vi "DateTimeStringToTimeString.vi"(10 "input string":string) -> (2 "concatenated string":string)   [LabVIEW 2012]
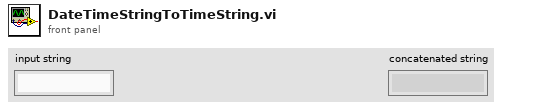
[diagram p1: front panel]
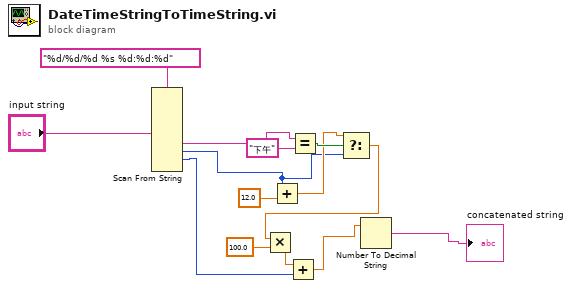
[diagram p0: block diagram]
diagram:
  n1 = Scan From String(format string="%d/%d/%d %s %d:%d:%d", input string="input string") -> (output 4=w12:string, output 5=w7:i32, output 6=w3:i32)  [unwired: 13 in, 3 out]
  n2 = Add(x=w7, y=12.0) -> (x+y=w8:dbl)
  n3 = Equal?(x=w12, y="下午") -> (x = y?=w10:bool)
  n4 = Select(t=w8, s=w10, f=w7) -> (s? t:f=w5:dbl)
  n5 = Multiply(x=w5, y=100.0) -> (x*y=w4:dbl)
  n6 = Add(x=w4, y=w3) -> (x+y=w2:dbl)
  n7 = Number To Decimal String(number=w2) -> (decimal integer string=→"concatenated string":string)  [unwired: 1 in]
